vi "StorageAcquireData.vi"() -> ()   [LabVIEW 2018]
panel:
  out "采集的数据数组":dbl[](array[numeric])
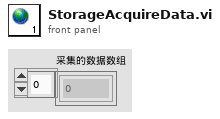
[diagram p1: front panel]
diagram:
